vi "DAQ Message Loop.vi"(8 "error in (no error)":errorcluster, 11 "Message Queues":T1) -> (0 "error out":errorcluster)   [LabVIEW 2018, in "DAQ.lvlib"]
doc: "Message loop for handling messages pertaining to the acquisition of data from the hardware."
uses:
  DAQ/DAQ.lvlib
  Main/Main Queue Cluster.ctl
  support/Message Queue/Message Cluster.ctl
  Acquisition State.ctl
  Hardware Configuration.ctl
  Task Cluster.ctl
  controls/Queue and Message Cluster.ctl
  support/Message Queue/Enqueue Message (Single).vi
  <vilib>/Utility/error.llb/Error Cluster From Error Code.vi
  <vilib>/ErrorRing/Error Ring.xnode
  DAQ/DAQ Write Folder/DAQ/DAQ Write.lvlib
  support/Message Queue/Message Queue.lvlib
  Acquisition Settings Dialog.vi
  support/Command Log VIs/Command Logging.lvlib
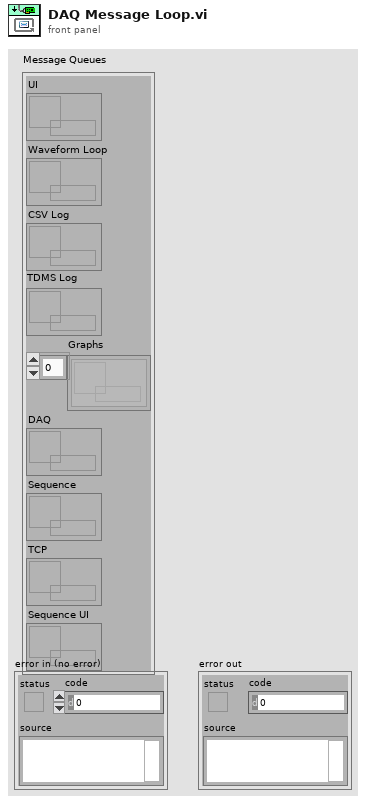
[diagram p1: front panel]
types:
  T1 = typedef "Main Queue Cluster.ctl" = cluster{"UI":refnum<queue>, "Waveform Loop":refnum<queue>, "CSV Log":refnum<queue>, "TDMS Log":refnum<queue>, "Graphs":refnum<queue>[], "DAQ":refnum<queue>, "Sequence":refnum<queue>, "TCP":refnum<queue>, "Sequence UI":refnum<queue>}
  T2 = typedef "DAQ.lvlib/Hardware Configuration.ctl" = cluster{"Tasks":T3[]}
  T3 = typedef "Task Cluster.ctl" = cluster{"DAQmx Task":refnum<k21>, "Read-Write Radio":enum32{"Read", "Write"}}
  T4 = typedef "DAQ Write.lvlib/Acquisition State.ctl" = enum16{"Idle", "Acquiring"}
  T5 = typedef "Queue and Message Cluster.ctl" = cluster{"return Message Queue":refnum<queue>, "Message":string, "Variant":variant}
  T6 = typedef "Message Queue.lvlib/Message Cluster.ctl" = cluster{"Message":string, "Message Data":variant}
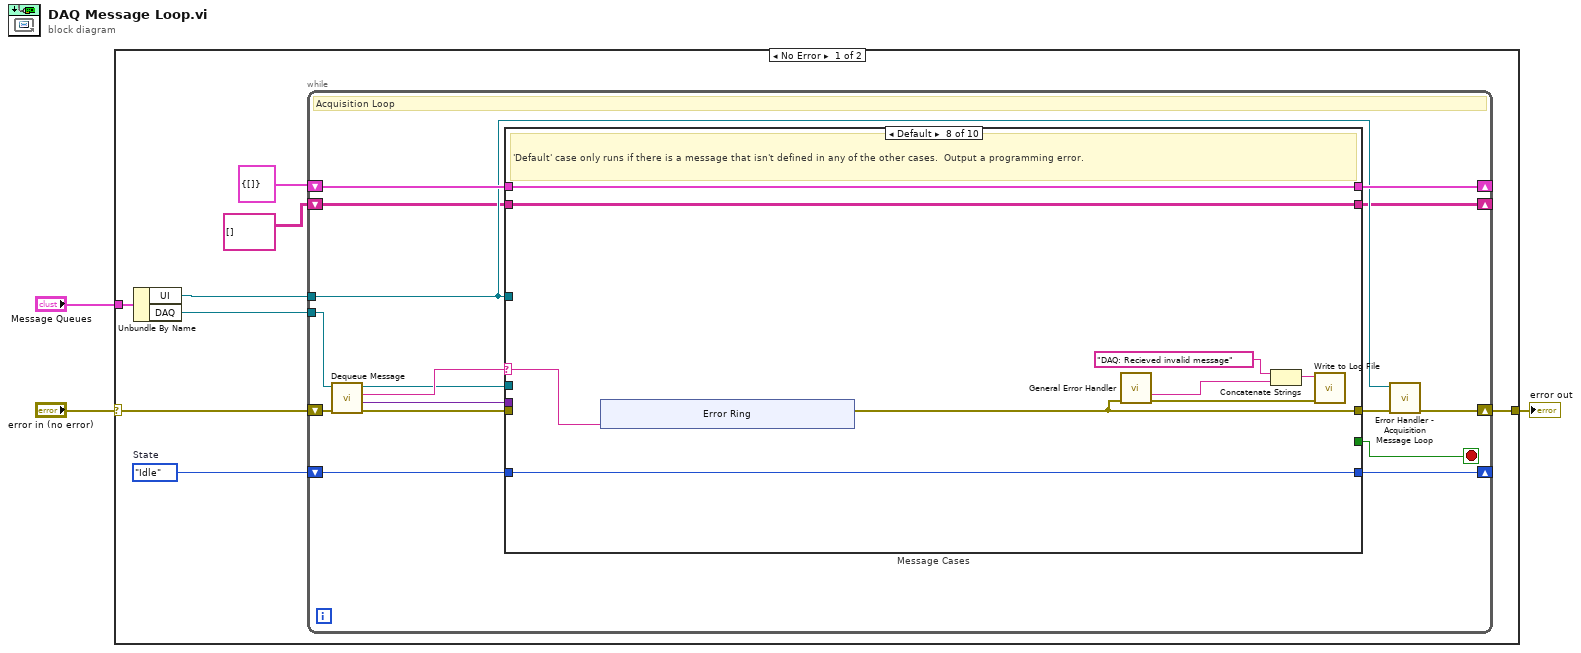
[diagram p0: block diagram]
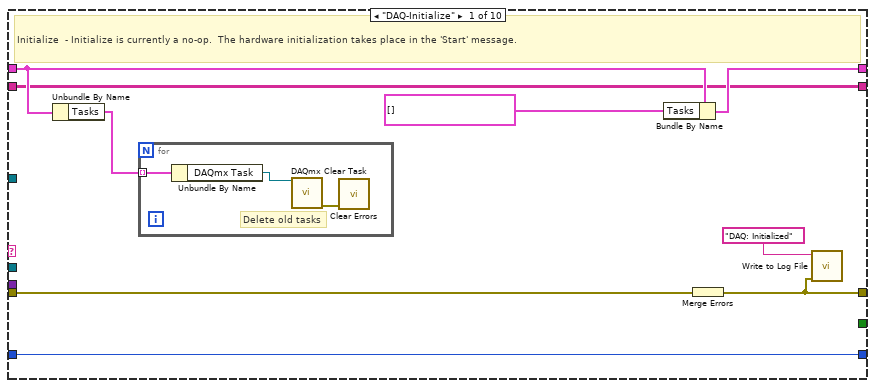
[diagram p2: hidden frame]
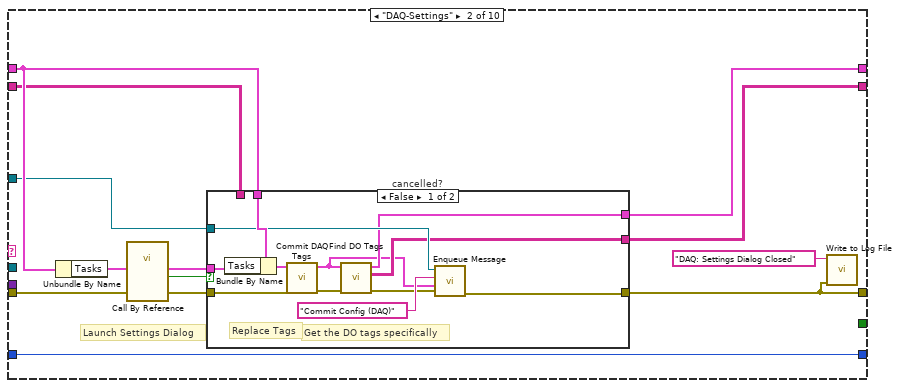
[diagram p3: hidden frame]
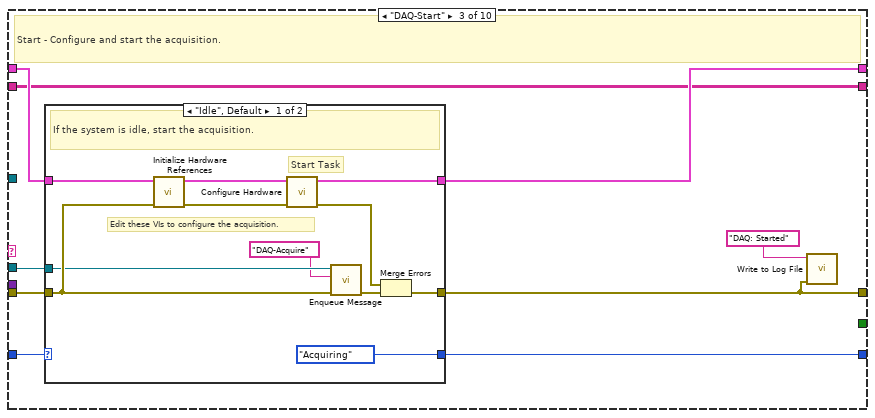
[diagram p5: hidden frame]
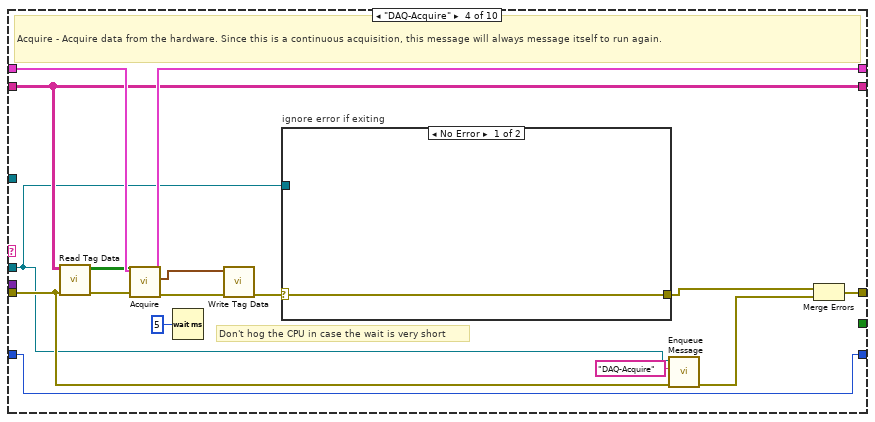
[diagram p7: hidden frame]
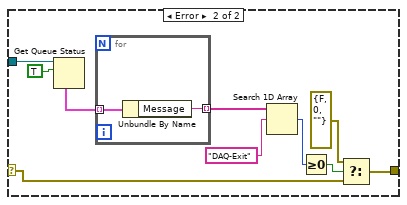
[diagram p8: hidden frame]
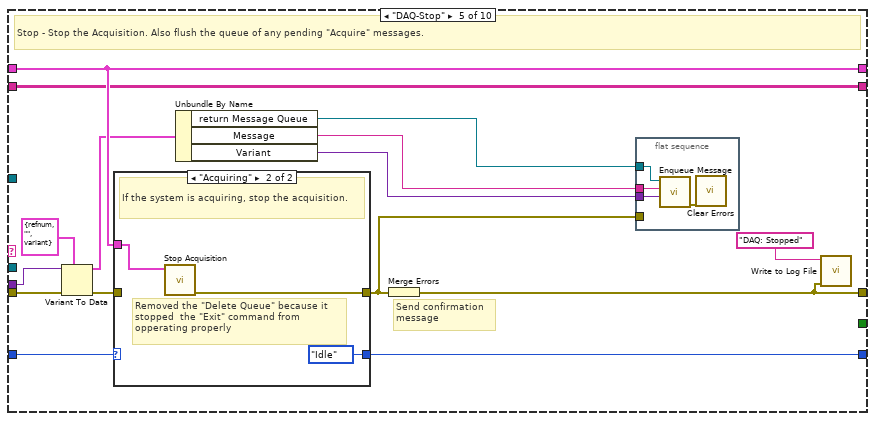
[diagram p9: hidden frame]
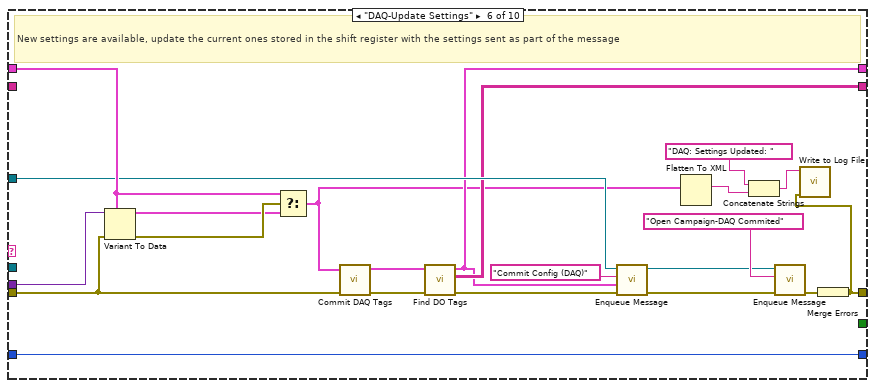
[diagram p11: hidden frame]
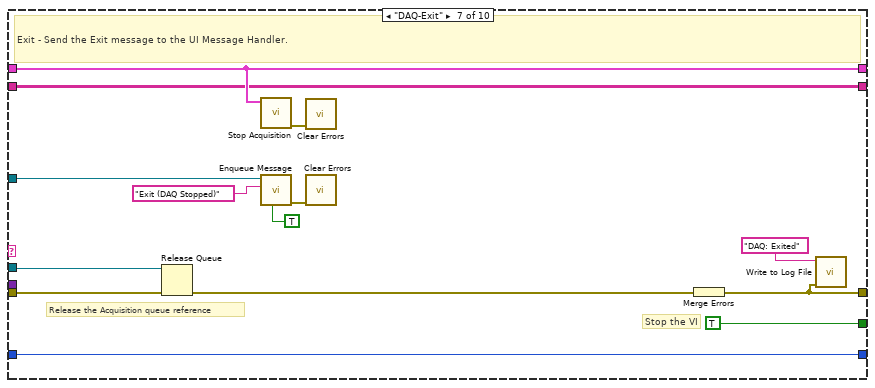
[diagram p12: hidden frame]
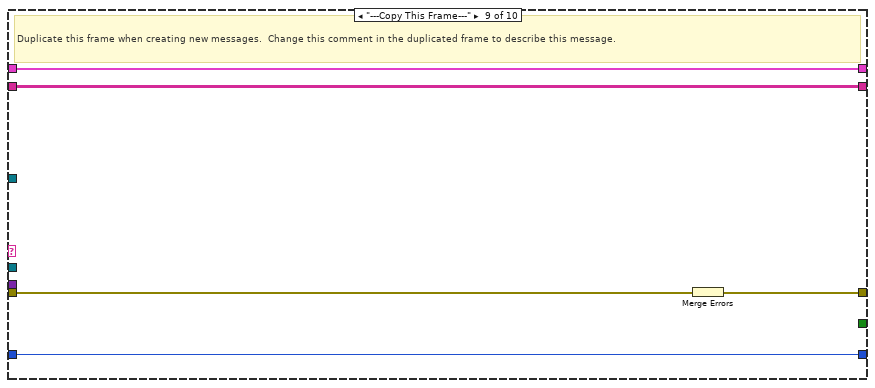
[diagram p13: hidden frame]
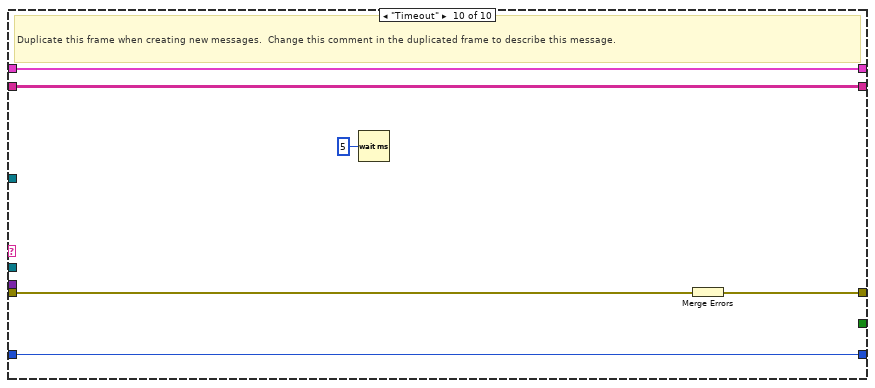
[diagram p14: hidden frame]
diagram:
  n1 = case shown="No Error" "error in (no error)" {
    selector: "error in (no error)" -> [w8 w207]
    tunnel: "Message Queues" -> [w11 _]
    tunnel: [w9 w207] -> w2
    frame No Error {
      w6 = Acquisition_State."Idle"  # State
      n2 = Unbundle By Name(w11) -> ("UI"=w7:refnum<queue>, "DAQ"=w10:refnum<queue>)
      n3 = while {
        tunnel: w10 -> [w21]
        shift-right: [w26] -> _
        shift-left: T2 {"Tasks"=[]} ("Data Cluster") -> [w27]
        shift-right: [w19] -> w9
        shift-left: w8 -> [w24]
        tunnel: w7 -> [w18]
        shift-right: [w16] -> _
        shift-left: w6 -> [w17]
        shift-right: [w15] -> _
        shift-left: string[][] [] ("Task D-O Channels") -> [w14]
        stop <- w25 stop-if-true
        # "Acquisition Loop"
        n4 = call "Dequeue Message.vi"("error in (no error)"=w24, "Message Queue"=w21) -> ("error out"=w13:errorcluster, "Message Data"=w22:variant, "Message"=w23:string, "dup Message Queue"=w12:refnum<queue>)  [unwired: 6 in]
        n5 = case "Message Cases" shown="Default" w23 {
          selector: w23 -> [_ _ _ _ _ _ _ w187 _ _]
          tunnel: w13 -> [w36 w50 w75 w96 w128 w160 w177 _ w200 w206]
          tunnel: [w28 w40 w68 w91 w120 w148 w166 w184 w198 w204] -> w20
          tunnel: w27 -> [w33 w48 w76 w105 w134 w162 w173 w188 w199 w205]
          tunnel: [w34 w47 w74 w106 w134 w149 w173 w188 w199 w205] -> w26
          tunnel: [_ _ _ _ _ _ TRUE _ _ _] -> w25
          tunnel: w22 -> [_ _ _ _ w130 w165 _ _ _ _]
          tunnel: w18 -> [_ w44 _ _ _ w155 w178 _ _ _]
          tunnel: w17 -> [w35 w52 w73 w104 w133 w161 w172 w186 w197 w203]
          tunnel: [w35 w52 w72 w104 w132 w161 w172 w186 w197 w203] -> w16
          tunnel: [w30 w43 w71 w93 w122 w150 w169 w185 w196 w202] -> w15
          tunnel: w14 -> [w30 w42 w71 w93 w122 _ w169 w185 w196 w202]
          tunnel: w12 -> [_ _ w70 w92 _ _ w168 _ _ _]
          frame "DAQ-Initialize" {
            # "Initialize  - Initialize is currently a no-op.  The hardware initialization takes place in the 'Start' message."
            n6 = Unbundle By Name(w33) -> ("Tasks"=w32:T3[])
            n7 = for {
              tunnel: w32 -> [w39] mode=indexing
              # "Delete old tasks"
              n8 = Unbundle By Name(w39) -> ("DAQmx Task"=w38:refnum<k21>)
              n9 = call <vilib>:"DAQmx Clear Task.vi"("task in"=w38) -> ("error out"=w37:errorcluster)  [unwired: 14 in]
              n10 = call <vilib>:"Clear Errors.vi"("error in (no error)"=w37) -> ()  [unwired: 5 in, 2 out]
            }
            n11 = Bundle By Name(cluster=w33, "Tasks"=T3[] []) -> (w34:T2)
            n12 = Merge Errors(w36) -> (w28:errorcluster)
            n13 = call "Write to Log File.vi"("error in"=w28, "text"="DAQ: Initialized") -> ()  [unwired: 9 in, 1 out]
          }
          frame "DAQ-Settings" {
            # "Launch Settings Dialog"
            n14 = Unbundle By Name(w48) -> ("Tasks"=w49:T3[])
            n15 = call-by-ref "?"("error in (no error)"=w50, "Tasks in"=w49) -> ("error out"=w45:errorcluster, "cancelled"=w46:bool, "Tasks out"=w51:T3[])  [unwired: 9 in, 2 out]
            n16 = case "cancelled?" shown="False" w46 {
              tunnel: w51 -> [w58 _]
              tunnel: w48 -> [w64 w67]
              tunnel: [w56 w67] -> w47
              tunnel: w45 -> [w62 w66]
              tunnel: [w60 w66] -> w40
              tunnel: w44 -> [w59 _]
              tunnel: [w57 w65] -> w43
              tunnel: w42 -> [_ w65]
              frame False {
                # "Get the DO tags specifically"
                # "Replace Tags"
                n17 = Bundle By Name(cluster=w64, "Tasks"=w58) -> (w63:T2)
                n18 = call "Commit DAQ Tags.vi"("error in (no error)"=w62, "DAQ State in"=w63) -> ("error out"=w55:errorcluster, "DAQ State out"=w53:T2)  [unwired: 8 in]
                n19 = call "Find DO Tags.vi"("error in (no error)"=w55, "DAQ State in"=w53) -> ("error out"=w54:errorcluster, "Task D-O Channels"=w57:string[][], "DAQ State out"=w56:T2)  [unwired: 7 in]
                n20 = call-poly "Enqueue Message.vi"("error in (no error)"=w54, "Message Data"=w53, "Message"="Commit Config (DAQ)", "Message Queue"=w59) -> ("error out"=w60:errorcluster)  [unwired: 6 in, 1 out]
              }
              frame True {
              }
            }
            n21 = call "Write to Log File.vi"("error in"=w40, "text"="DAQ: Settings Dialog Closed") -> ()  [unwired: 9 in, 1 out]
          }
          frame "DAQ-Start" {
            # "Start - Configure and start the acquisition."
            n22 = case shown="\"Idle\", Default" w73 {
              selector: w73 -> [_ w88]
              tunnel: [w87 w90] -> w68
              tunnel: w76 -> [w86 w89]
              tunnel: w75 -> [w85 w90]
              tunnel: w70 -> [w83 _]
              tunnel: [w79 w89] -> w74
              tunnel: [Acquisition_State."Acquiring" ("State") w88] -> w72
              frame "Idle", Default {
                # "Start Task"
                # "Edit these VIs to configure the acquisition."
                # "If the system is idle, start the acquisition."
                n23 = call "Initialize Hardware References.vi"("error in (no error)"=w85, "Hardware Resources in"=w86) -> ("error out"=w82:errorcluster, "Hardware Resources out"=w80:T2)  [unwired: 8 in]
                n24 = call "Configure Hardware.vi"("error in (no error)"=w82, "Hardware Resources in"=w80) -> ("error out"=w81:errorcluster, "Hardware Resources out"=w79:T2)  [unwired: 8 in]
                n25 = call-poly "Enqueue Message.vi"("error in (no error)"=w85, "Message"="DAQ-Acquire", "Message Queue"=w83) -> ("error out"=w84:errorcluster)  [unwired: 7 in, 1 out]
                n26 = Merge Errors(w81, w84) -> (w87:errorcluster)
              }
              frame "Acquiring" {
                # "The system is already acquiring. Ignore the \"Start\" message."
              }
            }
            n27 = call "Write to Log File.vi"("error in"=w68, "text"="DAQ: Started") -> ()  [unwired: 9 in, 1 out]
          }
          frame "DAQ-Acquire" {
            # "Don't hog the CPU in case the wait is very short"
            # "Acquire - Acquire data from the hardware. Since this is a continuous acquisition, this message will always message itself to run again."
            n28 = call "Read Tag Data.vi"("error in (no error)"=w96, "Task D-O Channels"=w93) -> ("error out"=w95:errorcluster, "Array"=w97:bool[][])  [unwired: 8 in]
            n29 = call "Acquire.vi"("error in (no error)"=w95, "Digital Write Status"=w97, "Hardware Resources in"=w105) -> ("error out"=w103:errorcluster, "data"=w102:waveform(dbl)[], "Hardware Resources out"=w106:T2)  [unwired: 6 in]
            n30 = Wait (ms)(milliseconds to wait=u32 5) -> ()  [unwired: 1 out]
            n31 = call "Write Tag Data.vi"("error in (no error)"=w103, "data"=w102) -> ("error out"=w100:errorcluster)  [unwired: 7 in, 2 out]
            n32 = case "ignore error if exiting" shown="No Error" w100 {
              selector: w100 -> [w107 w110]
              tunnel: w92 -> [_ w117]
              tunnel: [w107 w109] -> w99
              frame No Error {
              }
              frame Error {
                n33 = Get Queue Status(queue=w117, return elements? (F)=TRUE) -> (elements=w114:T6[])  [unwired: 1 in, 7 out]
                n34 = for {
                  tunnel: w114 -> [w119] mode=indexing
                  tunnel: [w118] -> w113 mode=indexing
                  n35 = Unbundle By Name(w119) -> ("Message"=w118:string)
                }
                n36 = Search 1D Array(1D array=w113, element="DAQ-Exit") -> (index of element=w112:i32)  [unwired: 1 in]
                n37 = Greater Or Equal To 0?(x=w112) -> (x >= 0?=w111:bool)
                n38 = Select(t=errorcluster {"status"=FALSE, "code"=0, "source"=""}, s=w111, f=w110) -> (s? t:f=w109:errorcluster)
              }
            }
            n39 = call-poly "Enqueue Message.vi"("error in (no error)"=w96, "Message"="DAQ-Acquire", "Message Queue"=w92) -> ("error out"=w98:errorcluster)  [unwired: 7 in, 1 out]
            n40 = Merge Errors(w99, w98) -> (w91:errorcluster)
          }
          frame "DAQ-Stop" {
            # "Send confirmation\nmessage"
            # "Stop - Stop the Acquisition. Also flush the queue of any pending \"Acquire\" messages."
            n41 = Variant To Data(error in=w128, type=T5 {"return Message Queue"=refnum, "Message"="", "Variant"=variant} ("Queue and Message"), Variant=w130) -> (data=w127:T5, error out=w129:errorcluster)
            n42 = case shown="\"Acquiring\"" w133 {
              selector: w133 -> [w140 _]
              tunnel: w129 -> [w139 _]
              tunnel: w134 -> [_ w143]
              tunnel: [w140 Acquisition_State."Idle" ("State")] -> w132
              tunnel: [w139 w141] -> w123
              frame "Idle", Default {
                # "The system is already idle. Ignore the \"Stop\" message."
              }
              frame "Acquiring" {
                # "Removed the \"Delete Queue\" because it\nstopped  the \"Exit\" command from \nopperating properly"
                # "If the system is acquiring, stop the acquisition."
                n43 = call "Stop Acquisition.vi"("Hardware Resources in"=w143) -> ("error out"=w141:errorcluster)  [unwired: 10 in]
              }
            }
            n44 = Unbundle By Name(w127) -> ("return Message Queue"=w126:refnum<queue>, "Message"=w125:string, "Variant"=w124:variant)
            n45 = Merge Errors(w123) -> (w120:errorcluster)
            n46 = flat-sequence {
              tunnel: w126 -> [w138]
              tunnel: w125 -> [w137]
              tunnel: w124 -> [w136]
              tunnel: w123 -> [_]
              frame #0 {
                n47 = call-poly "Enqueue Message.vi"("Message Data"=w136, "Message"=w137, "Message Queue"=w138) -> ("error out"=w135:errorcluster)  [unwired: 7 in, 1 out]
                n48 = call <vilib>:"Clear Errors.vi"("error in (no error)"=w135) -> ()  [unwired: 5 in, 2 out]
              }
            }
            n49 = call "Write to Log File.vi"("error in"=w120, "text"="DAQ: Stopped") -> ()  [unwired: 9 in, 1 out]
          }
          frame "DAQ-Update Settings" {
            # "New settings are available, update the current ones stored in the shift register with the settings sent as part of the message"
            n50 = Variant To Data(error in=w160, type=w162, Variant=w165) -> (data=w163:T2, error out=w164:errorcluster)
            n51 = Select(t=w162, s=w164, f=w163) -> (s? t:f=w144:T2)
            n52 = call "Commit DAQ Tags.vi"("error in (no error)"=w160, "DAQ State in"=w144) -> ("error out"=w157:errorcluster, "DAQ State out"=w151:T2)  [unwired: 8 in]
            n53 = call "Find DO Tags.vi"("error in (no error)"=w157, "DAQ State in"=w151) -> ("error out"=w154:errorcluster, "Task D-O Channels"=w150:string[][], "DAQ State out"=w149:T2)  [unwired: 7 in]
            n54 = call-poly "Enqueue Message.vi"("error in (no error)"=w154, "Message Data"=w149, "Message"="Commit Config (DAQ)", "Message Queue"=w155) -> ("error out"=w153:errorcluster, "dup Message Queue"=w152:refnum<queue>)  [unwired: 6 in]
            n55 = Flatten To XML(anything=w144) -> (xml string=w145:string)
            n56 = Concatenate Strings("DAQ: Settings Updated: " ("text"), w145) -> (w146:string)
            n57 = call-poly "Enqueue Message.vi"("error in (no error)"=w153, "Message"="Open Campaign-DAQ Commited", "Message Queue"=w152) -> ("error out"=w159:errorcluster)  [unwired: 7 in, 1 out]
            n58 = Merge Errors(w159) -> (w148:errorcluster)
            n59 = call "Write to Log File.vi"("error in"=w148, "text"=w146) -> ()  [unwired: 9 in, 1 out]
          }
          frame "DAQ-Exit" {
            # "Release the Acquisition queue reference"
            # "Stop the VI"
            # "Exit - Send the Exit message to the UI Message Handler."
            n60 = Release Queue(queue=w168, error in (no error)=w177) -> (error out=w174:errorcluster)  [unwired: 1 in, 2 out]
            n61 = call "Stop Acquisition.vi"("Hardware Resources in"=w173) -> ("error out"=w171:errorcluster)  [unwired: 10 in]
            n62 = call-poly "Enqueue Message.vi"("Priority Message? (F)"=TRUE, "Message"="Exit (DAQ Stopped)", "Message Queue"=w178) -> ("error out"=w170:errorcluster)  [unwired: 7 in, 1 out]
            n63 = call <vilib>:"Clear Errors.vi"("error in (no error)"=w171) -> ()  [unwired: 5 in, 2 out]
            n64 = call <vilib>:"Clear Errors.vi"("error in (no error)"=w170) -> ()  [unwired: 5 in, 2 out]
            n65 = Merge Errors(w174) -> (w166:errorcluster)
            n66 = call "Write to Log File.vi"("error in"=w166, "text"="DAQ: Exited") -> ()  [unwired: 9 in, 1 out]
          }
          frame Default {
            # "'Default' case only runs if there is a message that isn't defined in any of the other cases.  Output a programming error."
            n67 = xnode "Error Ring"("parameter 0"=w187) -> ("error out"=w184:errorcluster)
            n68 = call <vilib>:"General Error Handler.vi"("error in (no error)"=w184) -> ("message"=w181:string, "error out"=w180:errorcluster)  [unwired: 10 in, 3 out]
            n69 = Concatenate Strings("DAQ: Recieved invalid message" ("text"), w181) -> (w183:string)
            n70 = call "Write to Log File.vi"("error in"=w180, "text"=w183) -> ()  [unwired: 9 in, 1 out]
          }
          frame "---Copy This Frame---" {
            # "Duplicate this frame when creating new messages.  Change this comment in the duplicated frame to describe this message."
            n71 = Merge Errors(w200) -> (w198:errorcluster)
          }
          frame "Timeout" {
            # "Duplicate this frame when creating new messages.  Change this comment in the duplicated frame to describe this message."
            n72 = Wait (ms)(milliseconds to wait=u32 5) -> ()  [unwired: 1 out]
            n73 = Merge Errors(w206) -> (w204:errorcluster)
          }
        }
        n74 = call "Error Handler - Acquisition Message Loop.vi"("error in (no error)"=w20, "Message Queue"=w18) -> ("dup error in"=w19:errorcluster)  [unwired: 8 in, 1 out]
      }
    }
    frame Error {
    }
  }
  "error out" <- w2
